vi "Run Pattern Encoder.vi"(10 "Input":string, 11 "Pattern Parser":T1) -> (2 "error out":errorcluster, 3 "Encoded":string)   [LabVIEW 2020, in "Stream.lvlib" / "URLPattern.lvclass"]
uses:
  URLPattern.lvclass
  Pattern Parser.ctl
  Token.ctl
  Token Type.ctl
  Pattern Part.ctl
  Pattern Part Type.ctl
  Pattern Part Modifier.ctl
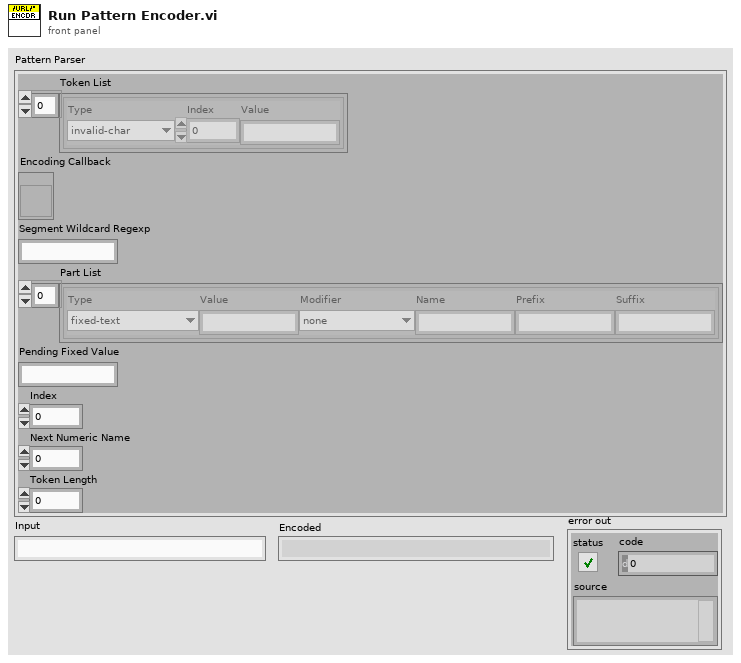
[diagram p1: front panel]
types:
  T1 = typedef "Stream.lvlib/URLPattern.lvclass/Pattern Parser.ctl" = cluster{"Token List":T2[], "Encoding Callback":refnum<vi>, "Segment Wildcard Regexp":string, "Part List":T4[], "Pending Fixed Value":string, "Index":i32, "Next Numeric Name":i32, "Token Length":i32}
  T2 = typedef "Stream.lvlib/URLPattern.lvclass/Token.ctl" = cluster{"Type":T3, "Index":i32, "Value":string}
  T3 = typedef "Stream.lvlib/URLPattern.lvclass/Token Type.ctl" = enum16{"invalid-char", "open", "close", "regexp", "name", "char", "escaped-char", "other-modifier", "asterisk", "end"}
  T4 = typedef "Stream.lvlib/URLPattern.lvclass/Pattern Part.ctl" = cluster{"Type":T5, "Value":string, "Modifier":T6, "Name":string, "Prefix":string, "Suffix":string}
  T5 = typedef "Stream.lvlib/URLPattern.lvclass/Pattern Part Type.ctl" = enum16{"fixed-text", "regexp", "segment-wildcard", "full-wildcard"}
  T6 = typedef "Stream.lvlib/URLPattern.lvclass/Pattern Part Modifier.ctl" = enum16{"none", "optional", "zero-or-more", "one-or-more"}
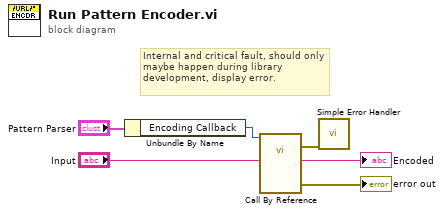
[diagram p0: block diagram]
diagram:
  # "Internal and critical fault, should only maybe happen during library development, display error."
  n1 = Unbundle By Name("Pattern Parser") -> ("Encoding Callback"=w4:refnum<vi>)
  n2 = call-by-ref "?"(reference=w4, "Value"="Input") -> (error out=w6:errorcluster, 0:"error out"=→"error out":errorcluster, "Canonicalized Protocol"=→"Encoded":string)  [unwired: 10 in, 1 out]
  n3 = call <vilib>:"Simple Error Handler.vi"("error in (no error)"=w6) -> ()  [unwired: 4 in, 5 out]
